vi "Remove View.vi"(8 "error in (no error)":errorcluster, 10 "View":string, 11 "GUI Container View Actor in":refnum<class "GUI Container Actor.lvclass">) -> (0 "error out":errorcluster, 3 "GUI Container View Actor out":refnum<class "GUI Container Actor.lvclass">)   [LabVIEW 2017, in "GUI Views.lvlib" / "GUI Container Actor.lvclass"]
uses:
  GUI Container Actor.lvclass
  GUI Container Actor.lvclass/GUI Container Actor.ctl
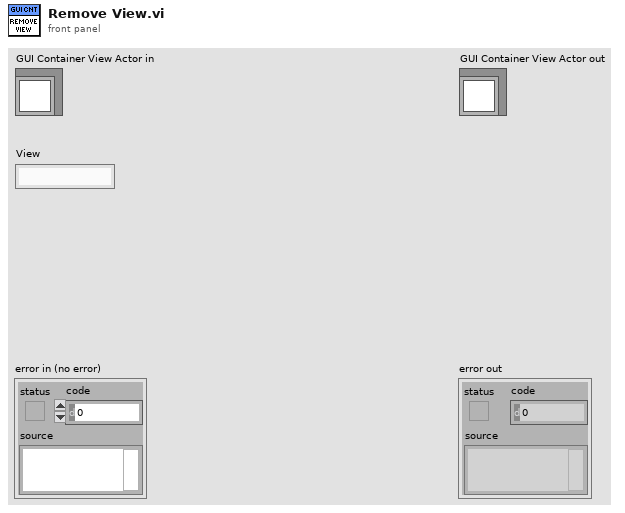
[diagram p1: front panel]
types:
  T1 = typedef "GUI Views.lvlib/GUI Container Actor.lvclass/View Status.ctl" = cluster{"View Details":T2, "Front Panel Statuses":T3[]}
  T2 = typedef "GUI Views.lvlib/GUI Container Actor.lvclass/View Details.ctl" = cluster{"Enqueuer":refnum<class "Message Enqueuer.lvclass">, "VI References":refnum<vi>[], "FP References":refnum<vi>[]}
  T3 = typedef "GUI Views.lvlib/GUI Container Actor.lvclass/FP Status.ctl" = cluster{"FP Open":bool, "Inserted in Subpanel":bool, "Subpanel":string}
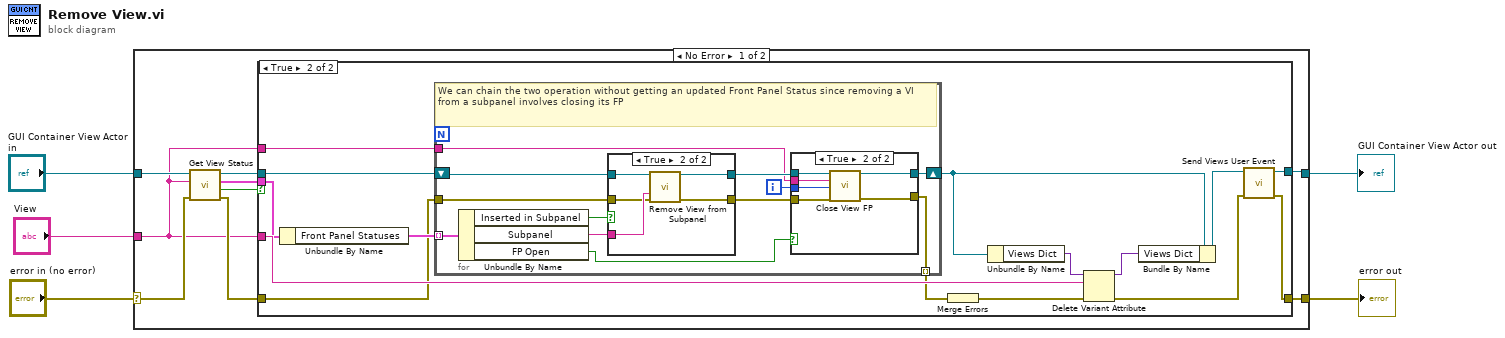
[diagram p0: block diagram]
diagram:
  n1 = case shown="No Error" "error in (no error)" {
    selector: "error in (no error)" -> [w11 w60]
    tunnel: [w13 w60] -> w4
    tunnel: [w14 w59] -> w2
    tunnel: "GUI Container View Actor in" -> [w12 w59]
    tunnel: "View" -> [w6 _]
    frame No Error {
      n2 = call "Get View Status.vi"("error in (no error)"=w11, "View"=w6, "GUI Container View Actor in"=w12) -> ("error out"=w10:errorcluster, "View Found"=w9:bool, "View Status"=w7:T1, "GUI Container View Actor out"=w8:refnum<class "GUI Container Actor.lvclass">)  [unwired: 5 in]
      n3 = case shown="True" w9 {
        tunnel: w10 -> [w15 w19]
        tunnel: [w16 w28] -> w14
        tunnel: [w15 w26] -> w13
        tunnel: w8 -> [w16 w23]
        tunnel: w6 -> [_ w25]
        tunnel: w7 -> [_ w24]
        tunnel: w6 -> [_ w17]
        frame False {
        }
        frame True {
          n4 = Unbundle By Name(w24) -> ("Front Panel Statuses"=w22:T3[])
          n5 = for {
            tunnel: w22 -> [w43] mode=indexing
            shift-right: [w39] -> w18
            shift-left: w23 -> [w41]
            tunnel: [w35] -> w21 mode=indexing
            tunnel: w19 -> [w34]
            tunnel: w17 -> [w32]
            i -> [w33]
            # "We can chain the two operation without getting an updated Front Panel Status since removing a VI from a subpanel involves closing its FP"
            n6 = Unbundle By Name(w43) -> ("Inserted in Subpanel"=w42:bool, "Subpanel"=w38:string, "FP Open"=w37:bool)
            n7 = case shown="True" w42 {
              tunnel: w41 -> [w53 w58]
              tunnel: [w53 w57] -> w40
              tunnel: w38 -> [_ w56]
              tunnel: [w52 w55] -> w36
              tunnel: w34 -> [w52 w54]
              frame False {
              }
              frame True {
                n8 = call "Remove View from Subpanel.vi"("GUI Container Actor in"=w58, "Subpanel"=w56, "error in (no error)"=w54) -> ("GUI Container Actor out"=w57:refnum<class "GUI Container Actor.lvclass">, "error out"=w55:errorcluster)  [unwired: 11 in]
              }
            }
            n9 = case shown="True" w37 {
              tunnel: w40 -> [w45 w51]
              tunnel: [w45 w50] -> w39
              tunnel: w36 -> [w44 w49]
              tunnel: [w44 w48] -> w35
              tunnel: w33 -> [_ w47]
              tunnel: w32 -> [_ w46]
              frame False {
              }
              frame True {
                n10 = call "Close View FP.vi"("GUI Container Actor in"=w51, "View"=w46, "View Hierarchy Level"=w47, "error in (no error)"=w49) -> ("GUI Container Actor out"=w50:refnum<class "GUI Container Actor.lvclass">, "error out"=w48:errorcluster)  [unwired: 10 in]
              }
            }
          }
          n11 = Merge Errors(w21) -> (w20:errorcluster)
          n12 = Unbundle By Name(w18) -> ("Views Dict"=w31:variant)
          n13 = Delete Variant Attribute(4:w20, 6:w25, 7:w31) -> (0:w27:errorcluster, 3:w30:variant)  [unwired: 1 out]
          n14 = Bundle By Name(cluster=w18, "Views Dict"=w30) -> (w29:refnum<class "GUI Container Actor.lvclass">)
          n15 = call "Send Views User Event.vi"("error in (no error)"=w27, "GUI Container Actor in"=w29) -> ("error out"=w26:errorcluster, "GUI Container Actor out"=w28:refnum<class "GUI Container Actor.lvclass">)  [unwired: 8 in]
        }
      }
    }
    frame Error {
    }
  }
  "error out" <- w4
  "GUI Container View Actor out" <- w2
